vi "Main.vi"() -> ()   [LabVIEW 2019]
uses:
  <vilib>/myRIO/Instrument Drivers/Onboard IO/SPI/typedefs/SPI User Configuration.ctl
  <vilib>/myRIO/Common/Instrument Driver Framework/myRIO v1.0/SPI/typedefs/SPI Clock Phase.ctl
  <vilib>/myRIO/Common/Instrument Driver Framework/myRIO v1.0/SPI/typedefs/SPI Clock Polarity.ctl
  <vilib>/myRIO/Common/Instrument Driver Framework/myRIO v1.0/SPI/typedefs/SPI Data Direction.ctl
  <vilib>/myRIO/Common/Instrument Driver Framework/myRIO v1.0/SPI/typedefs/SPI Frame Length.ctl
  <vilib>/myRIO/Instrument Drivers/Onboard IO/AO/typedefs/AO Reference.ctl
  <vilib>/myRIO/Common/Instrument Driver Framework/Utilities/typedefs/myRIO Generic Hardware Reference.ctl
  <vilib>/myRIO/Common/Instrument Driver Framework/Utilities/typedefs/Hardware Version Enum.ctl
  <vilib>/myRIO/Common/Instrument Driver Framework/Utilities/typedefs/myRIO v1.0 Reference.ctl
  <vilib>/myRIO/Common/Instrument Driver Framework/Utilities/typedefs/Generic FPGA Reference.ctl
  <vilib>/myRIO/Common/Instrument Driver Framework/myRIO v1.0/AO/typedefs/AO Channels List.ctl
  <vilib>/myRIO/Common/Instrument Driver Framework/myRIO v1.0/AO/typedefs/AO Channels Enum.ctl
  <vilib>/myRIO/Common/Instrument Driver Framework/Utilities/typedefs/Analog Scaling Constants List.ctl
  <vilib>/myRIO/Common/Instrument Driver Framework/Utilities/typedefs/Analog Scaling Constants.ctl
  <vilib>/userdefined/High Color/nirio_resource_hc.ctl
  <vilib>/myRIO/Instrument Drivers/Onboard IO/SPI/typedefs/SPI Reference.ctl
  <vilib>/myRIO/Common/Instrument Driver Framework/myRIO v1.0/SPI/typedefs/SPI Channels Enum.ctl
  <vilib>/myRIO/Instrument Drivers/Onboard IO/SPI/typedefs/SPI Configuration.ctl
  <vilib>/myRIO/Instrument Drivers/Onboard IO/DIO/typedefs/DIO Reference.ctl
  <vilib>/myRIO/Common/Instrument Driver Framework/myRIO v1.0/DIO/typedefs/DIO Channels List.ctl
  <vilib>/myRIO/Common/Instrument Driver Framework/myRIO v1.0/DIO/typedefs/DIO Channels Enum.ctl
  <vilib>/Platform/TimedLoop/XDataNode/timing_clust.ctl
  <vilib>/Platform/TimedLoop/XDataNode/nitl_modes.ctl
  <vilib>/Platform/TimedLoop/XDataNode/wakeup.ctl
  <vilib>/myRIO/Instrument Drivers/Onboard IO/AI/typedefs/AI Reference.ctl
  <vilib>/myRIO/Common/Instrument Driver Framework/myRIO v1.0/AI/typedefs/AI Channels List.ctl
  <vilib>/myRIO/Common/Instrument Driver Framework/myRIO v1.0/AI/typedefs/AI Channels Enum.ctl
  <vilib>/Analysis/3filter.llb/Filter Passband Type.ctl
  <vilib>/myRIO/Instrument Drivers/Onboard IO/PWM/typedefs/PWM Reference.ctl
  <vilib>/myRIO/Common/Instrument Driver Framework/myRIO v1.0/PWM/typedefs/PWM Channels Enum.ctl
  <vilib>/myRIO/Instrument Drivers/Onboard IO/PWM/typedefs/PWM Configuration.ctl
  <vilib>/myRIO/Common/Instrument Driver Framework/Utilities/vis/Is FPGA Ref Available.vi
  <vilib>/myRIO/Common/Instrument Driver Framework/myRIO v1.0/AO/vis/myRIO v1.1 Open AO.vi
  <vilib>/myRIO/Instrument Drivers/Onboard IO/AO/vis/Write.vi
  <vilib>/myRIO/Common/Instrument Driver Framework/myRIO v1.0/SPI/vis/myRIO v1.1 Open SPI.vi
  <vilib>/myRIO/Common/Instrument Driver Framework/myRIO v1.0/DIO/vis/myRIO v1.1 Open DIO.vi
  <vilib>/myRIO/Instrument Drivers/Onboard IO/DIO/vis/Write.vi
  <vilib>/myRIO/Common/Instrument Driver Framework/myRIO v1.0/AI/vis/myRIO v1.1 Open AI.vi
  <vilib>/myRIO/Instrument Drivers/Onboard IO/AI/vis/Read.vi
  <vilib>/myRIO/Common/Instrument Driver Framework/myRIO v1.0/PWM/vis/myRIO v1.1 Open PWM.vi
  <vilib>/myRIO/Instrument Drivers/Onboard IO/PWM/vis/Set Duty Cycle and Frequency.vi
  <vilib>/myRIO/Common/Instrument Driver Framework/Utilities/vis/Validate Channels.vi
  <vilib>/myRIO/Common/Instrument Driver Framework/myRIO v1.0/AO/vis/myRIO v1.0 Reserve AO.vi
  <vilib>/myRIO/Common/Instrument Driver Framework/myRIO v1.0/SPI/vis/myRIO v1.0 Reserve SPI.vi
  <vilib>/myRIO/Common/Instrument Driver Framework/myRIO v1.0/DIO/vis/myRIO v1.0 Reserve DIO.vi
  <vilib>/myRIO/Common/Instrument Driver Framework/myRIO v1.0/AI/vis/myRIO v1.0 Reserve AI.vi
  <vilib>/myRIO/Common/Instrument Driver Framework/myRIO v1.0/PWM/vis/myRIO v1.0 Reserve PWM.vi
  <vilib>/myRIO/Common/Instrument Driver Framework/myRIO v1.0/SPI/vis/myRIO v1.0 Close SPI.vi
  <vilib>/myRIO/Common/Instrument Driver Framework/myRIO v1.0/UART/vis/myRIO v1.0 Close UART.vi
  <vilib>/myRIO/Common/Instrument Driver Framework/myRIO v1.0/AO/vis/myRIO v1.0 Build MUX Configuration AO.vi
  <vilib>/myRIO/Common/Instrument Driver Framework/myRIO v1.0/Resource Manager/vis/myRIO v1.0 Reserve Channel List.vi
  <vilib>/myRIO/Common/Instrument Driver Framework/myRIO v1.0/SPI/vis/myRIO v1.0 Build MUX Configuration SPI.vi
  <vilib>/myRIO/Common/Instrument Driver Framework/myRIO v1.0/DIO/vis/myRIO v1.0 Build MUX Configuration DIO.vi
  <vilib>/myRIO/Common/Instrument Driver Framework/myRIO v1.0/AI/vis/myRIO v1.0 Build MUX Configuration AI.vi
  <vilib>/myRIO/Common/Instrument Driver Framework/myRIO v1.0/PWM/vis/myRIO v1.0 Build MUX Configuration PWM.vi
  <vilib>/myRIO/Common/Instrument Driver Framework/myRIO v1.0/SPI/vis/myRIO v1.0 Unreserve SPI.vi
  <vilib>/myRIO/Common/Instrument Driver Framework/myRIO v1.0/Resource Manager/vis/myRIO v1.0 Reserve Channel.vi
  <vilib>/myRIO/Common/Instrument Driver Framework/myRIO v1.0/Resource Manager/vis/myRIO v1.0 Unreserve Channel.vi
  <vilib>/myRIO/Common/Instrument Driver Framework/myRIO v1.0/Resource Manager/vis/myRIO v1.0 Create Configuration List.vi
  <vilib>/myRIO/Common/Instrument Driver Framework/myRIO v1.0/Resource Manager/vis/myRIO v1.0 Unreserve Channel List.vi
  <vilib>/myRIO/Common/Instrument Driver Framework/myRIO v1.0/Resource Manager/vis/myRIO v1.0 Build Mutex Name.vi
  <vilib>/Utility/VariantDataType/GetNumericInfo.vi
  <vilib>/Utility/error.llb/Error Cluster From Error Code.vi
  <vilib>/myRIO/Common/Instrument Driver Framework/myRIO v1.0/myRIO v1.1 Open.vi
  <vilib>/myRIO/Common/Instrument Driver Framework/Utilities/vis/IO Manager.vi
  <vilib>/myRIO/Common/Instrument Driver Framework/Utilities/vis/Configuration Manager.vi
  <vilib>/myRIO/Common/Instrument Driver Framework/myRIO v1.0/Resource Manager/vis/myRIO v1.0 Configure IO.vi
  <vilib>/myRIO/Common/Instrument Driver Framework/myRIO v1.0/myRIO v1.0 Close.vi
  <vilib>/myRIO/Common/Instrument Driver Framework/myRIO v1.0/DIO/vis/myRIO v1.0 Write DIO.vi
  <vilib>/myRIO/Common/Instrument Driver Framework/myRIO v1.0/SPI/vis/myRIO v1.0 Configure SPI.vi
  <vilib>/myRIO/Common/Instrument Driver Framework/myRIO v1.0/AO/vis/myRIO v1.0 Get Scaling Constants AO.vi
  <vilib>/myRIO/Common/Instrument Driver Framework/myRIO v1.0/AO/vis/myRIO v1.0 Write AO.vi
  <vilib>/myRIO/Common/Instrument Driver Framework/myRIO v1.0/AI/vis/myRIO v1.0 Get Scaling Constants AI.vi
  <vilib>/myRIO/Common/Instrument Driver Framework/myRIO v1.0/AI/vis/myRIO v1.0 Read AI.vi
  <vilib>/functionblocks/Edge Detection/One Shot Rising with Input/One Shot Rising with Input.vi
  <vilib>/myRIO/Common/Instrument Driver Framework/myRIO v1.0/PWM/vis/myRIO v1.0 Write PWM.vi
  <vilib>/myRIO/Common/Instrument Driver Framework/myRIO v1.0/SPI/vis/myRIO v1.0 Shutdown SPI.vi
  <vilib>/myRIO/Common/Instrument Driver Framework/Utilities/vis/FPGA Ref Manager.vi
  <vilib>/myRIO/Common/Instrument Driver Framework/myRIO v1.0/myRIO v1.0 Reset FPGA.vi
  <vilib>/myRIO/Common/Instrument Driver Framework/myRIO v1.0/IRQ/vis/myRIO v1.0 IRQ Info FGV.vi
  <vilib>/myRIO/Common/Instrument Driver Framework/myRIO v1.0/IRQ/vis/myRIO v1.0 Timer IRQ Info FGV.vi
  <vilib>/myRIO/Common/Instrument Driver Framework/myRIO v1.0/IRQ/vis/myRIO v1.0 ISR Agent.vi
  <vilib>/myRIO/Instrument Drivers/Utilities/vis/Reset Index.vi
  <vilib>/myRIO/Common/Instrument Driver Framework/myRIO v1.0/Resource Manager/vis/myRIO v1.0 Block Write Resource Manager.vi
  <vilib>/myRIO/Express VI/Onboard IO/DO/DO Express VI.xnode
  <vilib>/myRIO/Instrument Drivers/Onboard IO/DIO/vis/myRIO DIO Open.xnode
  <vilib>/myRIO/Instrument Drivers/Onboard IO/SPI/vis/myRIO SPI Open.xnode
  <vilib>/myRIO/Express VI/Onboard IO/AO/AO Express VI.xnode
  <vilib>/myRIO/Instrument Drivers/Onboard IO/AO/vis/myRIO AO Open.xnode
  <vilib>/Platform/TimedLoop/XDataNode/XDataNode.xnode
  <vilib>/myRIO/Express VI/Onboard IO/AI/AI Express VI.xnode
  <vilib>/myRIO/Instrument Drivers/Onboard IO/AI/vis/myRIO AI Open.xnode
  <vilib>/functionblocks/FB Core/FB Core.xnode
  <vilib>/regexp/Match Regular Expression.xnode
  <vilib>/myRIO/Express VI/Onboard IO/PWM/PWM Express VI.xnode
  <vilib>/myRIO/Instrument Drivers/Onboard IO/PWM/vis/myRIO PWM Open.xnode
  <vilib>/myRIO/Instrument Drivers/Utilities/Utilities.lvlib
  <vilib>/myRIO/Instrument Drivers/Onboard IO/SPI/SPI.lvlib
  <vilib>/myRIO/Instrument Drivers/Onboard IO/AI/AI.lvlib
  <vilib>/Platform/TimedLoop/XDataNode/XDNodeRunTimeDep.lvlib
  <vilib>/myRIO/Instrument Drivers/Onboard IO/DIO/DIO.lvlib
  <vilib>/myRIO/Instrument Drivers/Onboard IO/PWM/PWM.lvlib
  <vilib>/myRIO/Instrument Drivers/Onboard IO/AO/AO.lvlib
  <vilib>/functionblocks/NI_FunctionBlock Libraries.lvlib
  <vilib>/ptbypt/NI_PtbyPt.lvlib
  <vilib>/Analysis/NI_AALBase.lvlib
panel:
  in  "Leg Length":dbl=1.0
  out "Speed":cluster{"Numeric":dbl, dbl}(graph)
  in  "Controller":enum16{"ML", "TBE"}(ring)
  out "size(s)":i32
  in  "SEND DATA !!\nLETS GO!":bool
  out "R.FSR":bool
  out "L.FSR":bool
  out "True Walking Speed":dbl=0.1 format="%#_13g"
  out "Assistant Profile":cluster{dbl, dbl}(graph)
  in  "Torque GO!":bool
  out "Trunk IMU":T1(graph)
  out "Right IMU":T1(graph)
  in  "Body Weight":dbl
  in  "Hip Angle Init":bool
  out "SYNC":bool
  in  "Assist":bool
  out "L.Limit":bool
  out "R.Limit":bool
  out "Left Torque":T2(graph)
  in  "Saving File Name":string
  out "Hip Angle":cluster{dbl, dbl}(graph)
  out "Right Torque":T3(graph)
  out "Run Time":dbl
  in  "Motor Enable":bool
  out "Loop Time":u32
  in  "STOP":bool
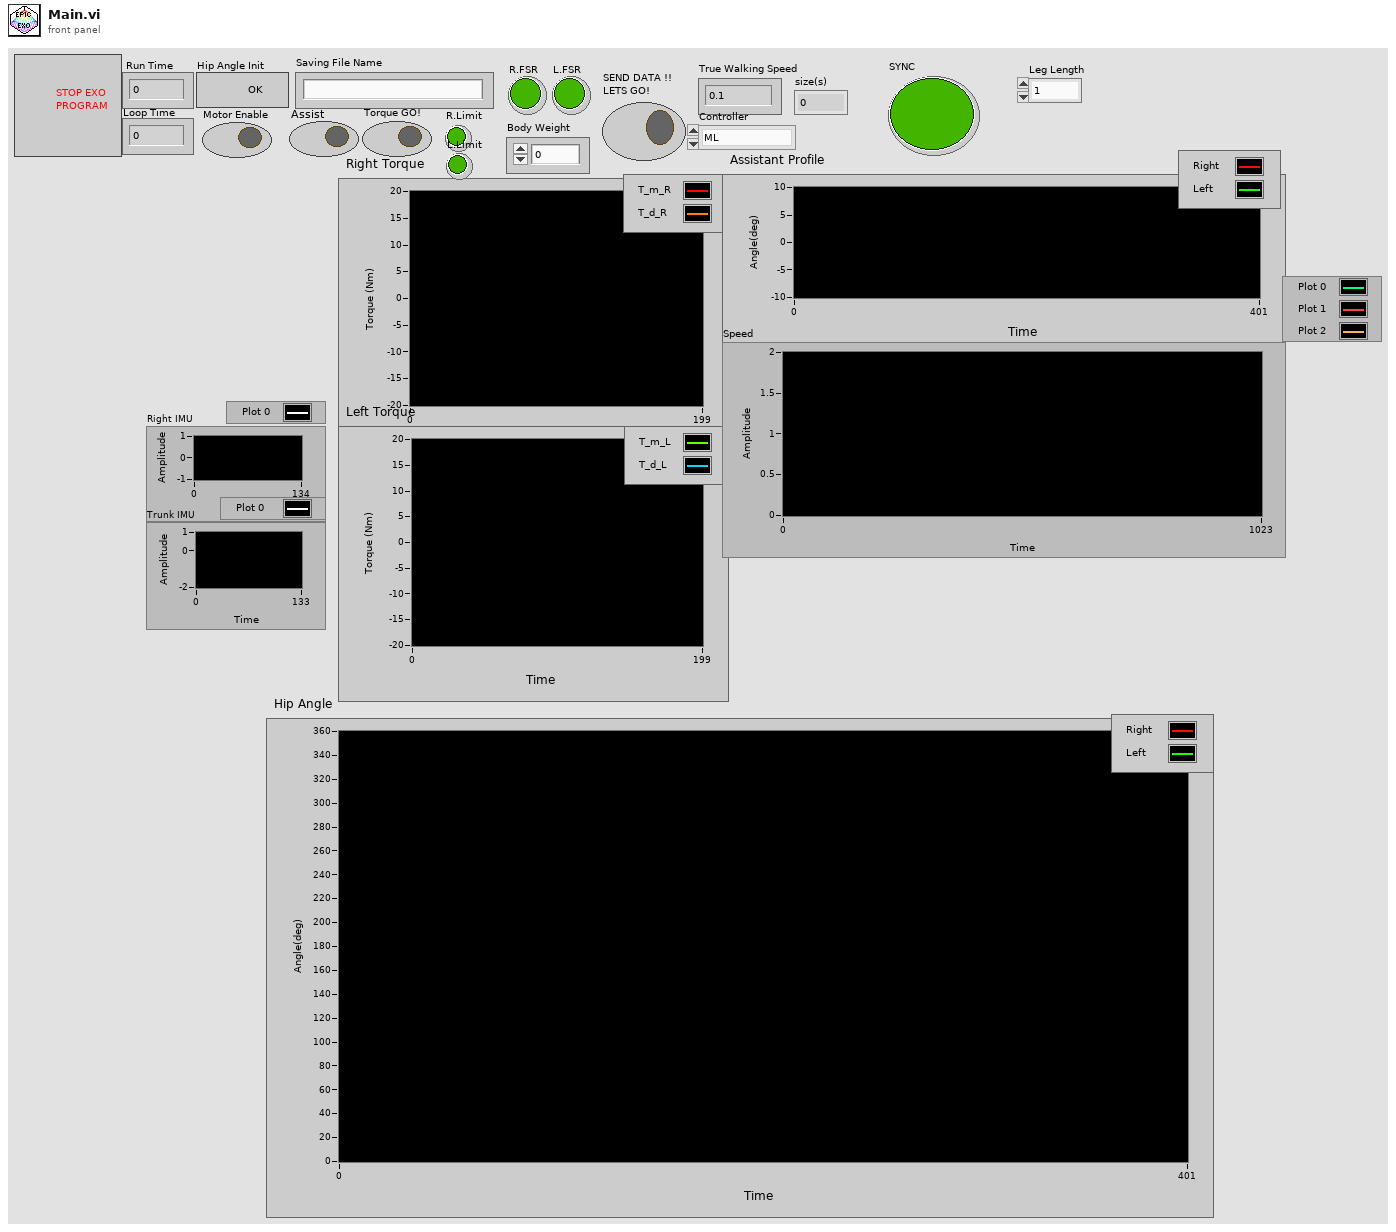
[diagram p1: front panel]
types:
  T1 = cluster{"[0]":dbl, "[1]":dbl, "[2]":dbl, "[3]":dbl, "[4]":dbl, "[5]":dbl, "[6]":dbl, "[7]":dbl, "[8]":dbl}
  T2 = cluster{"Left Torque":dbl, "Left Desired Torque":dbl}
  T3 = cluster{"Right Torque in":dbl, "Right Torque Desired":dbl}
  T4 = typedef "SPI.lvlib/SPI User Configuration.ctl" = cluster{"Frequency [Hz]":dbl, "Clock Phase":T5, "Clock Polarity":T6, "Data Direction":T7, "Frame Length":T8}
  T5 = typedef "SPI Clock Phase.ctl" = enum8{"Leading", "Trailing"}
  T6 = typedef "SPI Clock Polarity.ctl" = enum8{"Low", "High"}
  T7 = typedef "SPI Data Direction.ctl" = enum8{"Most significant bit first", "Least significant bit first"}
  T8 = typedef "SPI Frame Length.ctl" = u8
  T9 = typedef "AO.lvlib/AO Reference.ctl" = cluster{"myRIO Reference":T10, "AO Channel List":T14, "AO Scaling Constant List":T16}
  T10 = typedef "myRIO Generic Hardware Reference.ctl" = cluster{"myRIO Model":T11, "myRIO Hardware Reference":T12}
  T11 = typedef "Hardware Version Enum.ctl" = enum16{"Unknown", "myRIO-1900", "myRIO-1950", "roboRIO", "NI ELVIS RIO CM", "ELVIS III"}
  T12 = typedef "myRIO v1.0 Reference.ctl" = cluster{"Generic FPGA Reference":T13, "Allow multiple opens":bool}
  T13 = typedef "Generic FPGA Reference.ctl" = refnum<k20>
  T14 = typedef "AO Channels List.ctl" = T15[]
  T15 = typedef "AO Channels Enum.ctl" = enum16{"Not Connected", "AudioOut/Left", "AudioOut/Right", "C/AO0", "C/AO1", "A/AO0", "A/AO1", "B/AO0", "B/AO1"}
  T16 = typedef "Analog Scaling Constants List.ctl" = T17[]
  T17 = typedef "Analog Scaling Constants.ctl" = cluster{"LSB Weight (Volts)":dbl, "Offset (Volts)":dbl, "Signed?":bool}
  T18 = typedef "nirio_resource_hc.ctl" = tag
  T19 = typedef "DIO.lvlib/DIO Reference.ctl" = cluster{"myRIO Reference":T10, "DIO Channels List":T20}
  T20 = typedef "DIO Channels List.ctl" = T21[]
  T21 = typedef "DIO Channels Enum.ctl" = enum16{"Not Connected", "C/DIO0", "C/DIO1", "C/DIO2", "C/DIO3", "C/DIO4", "C/DIO5", "C/DIO6", "C/DIO7", "A/DIO0", "A/DIO1", "A/DIO2", "A/DIO3", "A/DIO4", "A/DIO5", "A/DIO6", "A/DIO7", "A/DIO8", "A/DIO9", "A/DIO10", "A/DIO11", "A/DIO12", "A/DIO13", "A/DIO14", "A/DIO15", "A/DIO16", "A/DIO17", "A/DIO18", "A/DIO19", "B/DIO0", "B/DIO1", "B/DIO2", "B/DIO3", "B/DIO4", "B/DIO5", "B/DIO6", "B/DIO7", "B/DIO8", "B/DIO9", "B/DIO10", "B/DIO11", "B/DIO12", "B/DIO13", "B/DIO14", "B/DIO15", "B/DIO16", "B/DIO17", "B/DIO18", "B/DIO19", "LED0", "LED1", "LED2", "LED3", "Button0", "DIO/DIO0", "DIO/DIO1", "DIO/DIO2", "DIO/DIO3", "DIO/DIO4", "DIO/DIO5", "DIO/DIO6", "DIO/DIO7", "DIO/DIO8", "DIO/DIO9", "SPI/CS0", "SPI/CS1", "SPI/CS2", "SPI/CS3", "LED RADIO (Green)", "LED RADIO (Red)", "LED COMM (Green)", "LED COMM (Red)", "LED MODE (Green)", "LED MODE (Red)"}
  T22 = typedef "AI.lvlib/AI Reference.ctl" = cluster{"myRIO Reference":T10, "AI Channels List":T23, "AI Scaling Constants List":T16}
  T23 = typedef "AI Channels List.ctl" = T24[]
  T24 = typedef "AI Channels Enum.ctl" = enum16{"Not Connected", "AudioIn/Left", "AudioIn/Right", "C/AI0", "C/AI1", "A/AI0", "A/AI1", "A/AI2", "A/AI3", "A/AI4", "A/AI5", "A/AI6", "A/AI7", "B/AI0", "B/AI1", "B/AI2", "B/AI3", "B/AI4", "B/AI5", "B/AI6", "B/AI7", "AI/AI0", "AI/AI1", "AI/AI2", "AI/AI3", "A/AI0 (DIFF)", "A/AI1 (DIFF)", "A/AI2 (DIFF)", "A/AI3 (DIFF)", "B/AI0 (DIFF)", "B/AI1 (DIFF)", "B/AI2 (DIFF)", "B/AI3 (DIFF)"}
  T25 = typedef "XDNodeRunTimeDep.lvlib/timing_clust.ctl" = cluster{"Expected End [f-1]":u64, "Actual End [f-1]":u64, "Finished Late? [f-1]":bool, "Expected End [i-1]":u64, "Actual End [i-1]":u64, "Finished Late? [i-1]":bool, "Expected Start [i]":u64, "Actual Start [i]":u64, "Expected Start [f]":u64, "Actual Start [f]":u64, "Source Name":string, "Structure Name":string, "Period":i64, "Deadline":i64, "Offset":i64, "Start":i64, "Priority":i32, "Timeout":i32, "Mode":T26, "Wakeup Reason":T27, "Error":errorcluster, "Source Type":string, "Secondary Source Type":string, "Global End Time":u64, "Global Start Time":u64, "Frame Duration":u64, "Iteration Duration":u64, "Assigned CPU":i32, "I/O Scan Engine Mode":u32}
  T26 = typedef "XDNodeRunTimeDep.lvlib/nitl_modes.ctl" = enum32{"No Change", "Process missed periods, maintain original phase", "Discard missed periods, maintain original phase", "Process missed periods, ignore original phase", "Discard missed periods, ignore original phase"}
  T27 = typedef "XDNodeRunTimeDep.lvlib/wakeup.ctl" = enum32{"Normal", "Aborted", "Asynchronous wakeup", "Timing source error", "Timed loop error", "Timeout"}
  T28 = enum16{"Standard", "Buffered", "CRLF", "Immediate"}
  T29 = typedef "NI_AALBase.lvlib/Filter Passband Type.ctl" = enum32{"Lowpass", "Highpass", "Bandpass", "Bandstop"}
  T30 = typedef "PWM.lvlib/PWM Reference.ctl" = cluster{"myRIO Reference":T10, "PWM Channels Enum":T31, "PWM Configuration":T32}
  T31 = typedef "PWM Channels Enum.ctl" = enum16{"Not Connected", "C/PWM0", "C/PWM1", "A/PWM0", "A/PWM1", "A/PWM2", "A/PWM3", "A/PWM4", "A/PWM5", "A/PWM6", "A/PWM7", "A/PWM8", "A/PWM9", "A/PWM10", "A/PWM11", "A/PWM12", "A/PWM13", "A/PWM14", "A/PWM15", "A/PWM16", "A/PWM17", "A/PWM18", "A/PWM19", "B/PWM0", "B/PWM1", "B/PWM2", "B/PWM3", "B/PWM4", "B/PWM5", "B/PWM6", "B/PWM7", "B/PWM8", "B/PWM9", "B/PWM10", "B/PWM11", "B/PWM12", "B/PWM13", "B/PWM14", "B/PWM15", "B/PWM16", "B/PWM17", "B/PWM18", "B/PWM19", "PWM/PWM0", "PWM/PWM1", "PWM/PWM2", "PWM/PWM3", "PWM/PWM4", "PWM/PWM5", "PWM/PWM6", "PWM/PWM7", "PWM/PWM8", "PWM/PWM9"}
  T32 = typedef "PWM.lvlib/PWM Configuration.ctl" = cluster{"Frequency":dbl, "Duty Cycle":dbl}
  T33 = typedef "SPI.lvlib/SPI Reference.ctl" = cluster{"myRIO Reference":T10, "SPI Channels Enum":T34, "SPI Configuration":T35}
  T34 = typedef "SPI Channels Enum.ctl" = enum16{"Not Connected", "A/SPI", "B/SPI", "SPI/SPI"}
  T35 = typedef "SPI.lvlib/SPI Configuration.ctl" = cluster{"Frequency [Hz]":dbl, "Clock Phase":T5, "Clock Polarity":T6, "Data Direction":T7, "Frame Length":T8}
  T36 = cluster{"Torque Output":dbl, "Torque Output":dbl}
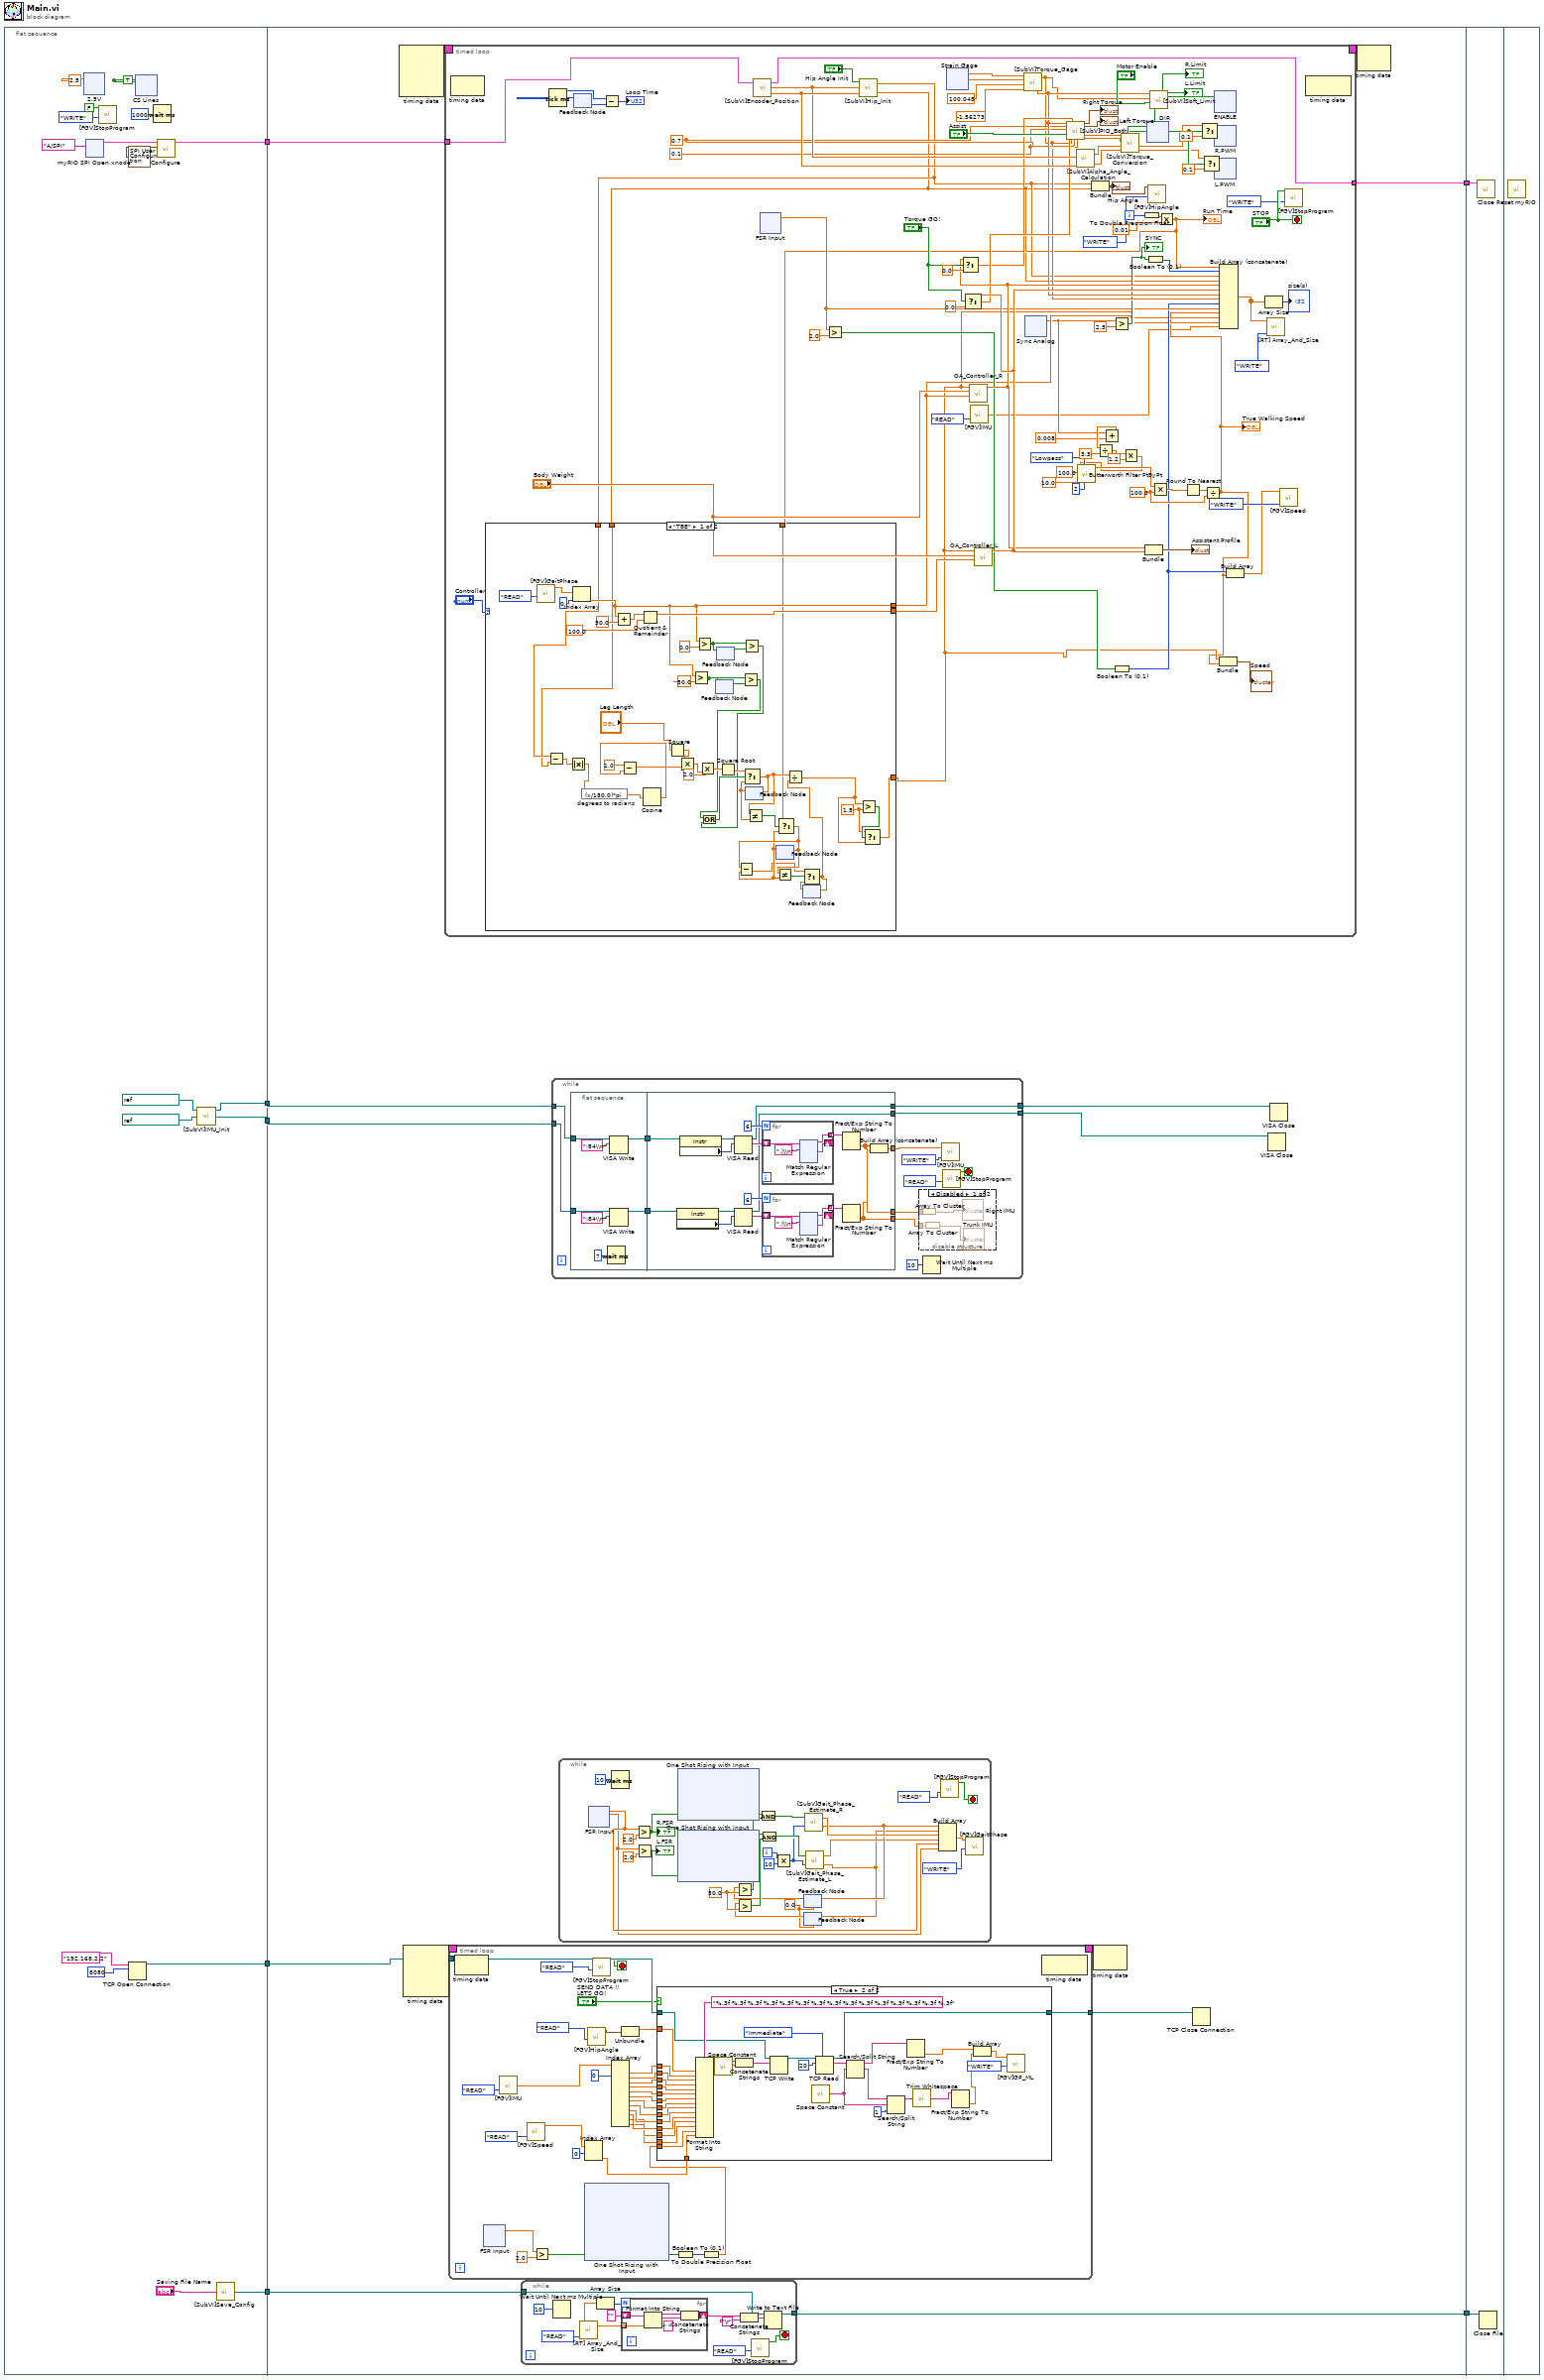
[diagram p0: block diagram]
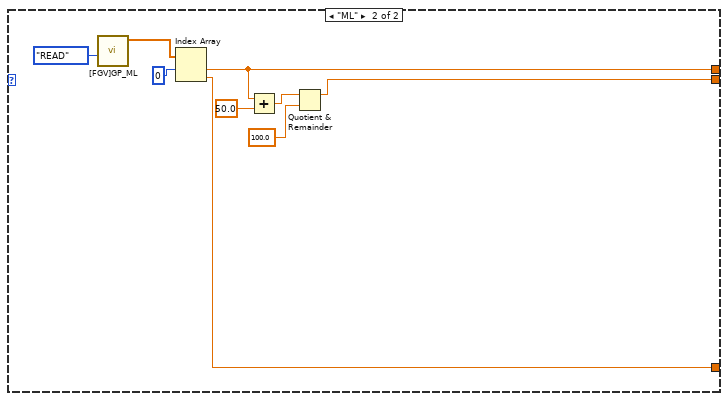
[diagram p4: hidden frame]
diagram:
  n1 = flat-sequence {
    tunnel: [w20] -> w7
    tunnel: [w18] -> w4
    tunnel: [w9] -> w3
    tunnel: [w8] -> w2
    tunnel: [w12] -> w1
    tunnel: w7 -> [w126]
    tunnel: [w125] -> w6
    tunnel: [w124] -> w5
    tunnel: w4 -> [w123]
    tunnel: w3 -> [w120]
    tunnel: w2 -> [w119]
    tunnel: w1 -> [w117]
    tunnel: w6 -> [w1117]
    tunnel: w5 -> [w1116]
    frame #0 {
      w16 = TRUE ("A/DIO2 (Pin 15)")
      n2 = xnode "2.5V"("2.5V (B/AO0 (Pin 2))"=2.5 ("2.5V (A/AO0 (Pin 2))")) -> ()  [unwired: 1 in, 1 out]
      n3 = xnode "myRIO SPI Open.xnode"("Channel Name"=tag "A/SPI") -> ("SPI Ref Out"=w23:T33)  [unwired: 2 in, 1 out]
      n4 = call "[FGV]StopProgram.vi"("Select"=enum16{"READ", "WRITE"}."WRITE", "Flag In"=FALSE) -> ()  [unwired: 9 in, 1 out]
      n5 = TCP Open Connection(address="192.168.2.2", remote port or service name=u16 8080) -> (connection ID=w12:refnum<k5>)  [unwired: 3 in, 1 out]
      n6 = xnode "CS Lines"("cs1 (A/DIO14 (Pin 32))"=w16, "cs2 (A/DIO15 (Pin 34))"=w16) -> ()  [unwired: 1 in, 1 out]
      n7 = Wait (ms)(milliseconds to wait=u32 1000) -> ()  [unwired: 1 out]
      n8 = call <vilib>:"Configure.vi"("SPI User Configuration"=T4 {"Frequency [Hz]"=4000000.0, "Clock Phase"=enum."Trailing", "Clock Polarity"=enum."Low", "Data Direction"=enum."Most significant bit first", "Frame Length"=8}, "SPI Ref In"=w23) -> ("SPI Ref Out"=w20:T33)  [unwired: 8 in, 1 out]
      n9 = call "[SubVI]IMU_Init.vi"("IMU Left"=refnum<visa-resource-name> "ASRL4::INSTR" ("VISA resource name"), "IMU Thigh"=refnum<visa-resource-name> "ASRL5::INSTR" ("VISA resource name")) -> ("IMU Left Out"=w8:refnum<visa-resource-name>, "IMU Right Out"=w9:refnum<visa-resource-name>)  [unwired: 1 in, 1 out]
      n10 = call "[SubVI]Save_Config.vi"("Saving File Name"="Saving File Name") -> ("Byte Stream File out"=w18:refnum<file>)
    }
    frame #1 {
      n11 = node-c288() -> (w128:T25)  [unwired: 4 in]
      n12 = node-c288() -> (w116:T25)  [unwired: 4 in]
      n13 = timed-loop {
        timing: w128 -> [_]
        timing-out: [_] -> w127
        tunnel: w126 -> [w781]
        tunnel: [w799] -> w125
        i -> [w776]
        stop <- "STOP" stop-if-true
        w751 = 100.0 ("y")
        w757 = 0.7 ("kp_right")
        w756 = 0.1 ("kd_right")
        n14 = node-c288() -> ()  [unwired: 1 in, 1 out]
        n15 = Tick Count (ms)() -> (millisecond timer value=w795:u32)
        n16 = feedback-in #1(w795) -> ()
        n17 = feedback #1() -> (w794:u32)  [unwired: 1 in]
        n18 = Subtract(x=w795, y=w794) -> (x-y=→"Loop Time":u32)
        n19 = call "[SubVI]Encoder_Position.vi"("SPI Reference In in"=w781) -> ("Left Theta"=w767:dbl, "Right Theta"=w766:dbl, "SPI Reference In out"=w799:T33)  [unwired: 2 out]
        n20 = xnode "FSR Input"() -> ("FSR 1 - Right (B/AI0 (Pin 3))"=w738:dbl)  [unwired: 1 in, 2 out]
        n21 = Greater?(x=w738, y=2.0) -> (0:w736:bool)
        n22 = call "[SubVI]Hip_Init.vi"("Left Theta"=w767, "Right Theta"=w766, "Hip Init"="Hip Angle Init") -> ("Left Hip"=w730:dbl, "Right Hip"=w731:dbl)
        n23 = xnode "Strain Gage"() -> ("Right (B/AI2 (Pin 7))"=w788:dbl, "Left (B/AI3 (Pin 9))"=w787:dbl)  [unwired: 1 in, 1 out]
        n24 = call "[FGV]IMU.vi"("Select"=enum16{"READ", "WRITE"}."READ") -> ("IMU Out"=w714:dbl[])  [unwired: 1 in]
        n25 = call "[SubVI]Torque_Gage.vi"("Left Offset"=-1.56273 ("Right Offset"), "Right Offset"=100.045, "Left Input"=w787, "Right Input"=w788) -> ("Right Torque"=w758:dbl, "Left Torque"=w754:dbl)
        n26 = xnode "Sync Analog"() -> ("A/AI0 (Pin 3)"=w720:dbl)  [unwired: 1 in, 1 out]
        n27 = call "[SubVI]Alpha_Angle_Calculation.vi"("Left Theta"=w767, "Right Theta"=w766) -> ("Left Alpha"=w764:dbl, "Right Alpha"=w765:dbl)  [unwired: 2 in]
        n28 = Bundle("Right Hip"=w731, "Left Hip"=w730) -> (w769:cluster{"Right Hip":dbl, "Left Hip":dbl})  [unwired: 1 in]
        "Hip Angle" <- w769
        n29 = Add(x=w720, y=0.008) -> (x+y=w721:dbl)
        n30 = Divide(x=w721, y=3.3) -> (x/y=w723:dbl)
        n31 = Greater?(x=w720, y=2.5) -> (0:w749:bool)
        "SYNC" <- w749
        n32 = Boolean To (0,1)(Boolean=w736) -> (0, 1=w735:i16)
        n33 = Multiply(x=w723, y=1.2) -> (x*y=w719:dbl)
        n34 = call <vilib>:"Butterworth Filter PtByPt.vi"("order"=2, "filter type"=Filter_Passband_Type."Lowpass", "low cutoff freq: fl"=10.0, "sampling freq: fs"=100.0, "x"=w719) -> ("Filtered x"=w725:dbl)  [unwired: 4 in, 1 out]
        n35 = To Double Precision Float(number=w776) -> (double precision float=w790:dbl)
        n36 = Boolean To (0,1)(Boolean=w749) -> (0, 1=w792:i16)
        n37 = call "[FGV]HipAngle.vi"("Select"=enum16{"READ", "WRITE"}."WRITE", "Hip In"=w769) -> ()  [unwired: 9 in, 1 out]
        n38 = call "[SubVI]Soft_Limit.vi"("Motor Enable in"="Motor Enable", "Left Torque"=w754, "Right Torque"=w758) -> ("PWM out"=w783:bool, "ENA out"=w782:bool, "L.SLimit"=→"L.Limit":bool, "R.SLimit"=→"R.Limit":bool)  [unwired: 1 in]
        n39 = Multiply(x=w725, y=w751) -> (x*y=w753:dbl)
        n40 = Multiply(x=w790, y=0.01) -> (x*y=w732:dbl)
        "Run Time" <- w732
        n41 = case shown="\"TBE\"" "Controller" {
          tunnel: [w839 w850] -> w733
          tunnel: [w842 w851] -> w734
          tunnel: w732 -> [w810 _]
          tunnel: [w804 w849] -> w716
          tunnel: w731 -> [w809 _]
          tunnel: w730 -> [w808 _]
          frame "TBE" {
            w806 = 1.5 ("y")
            n42 = call "[FGV]GaitPhase.vi"("Select"=enum16{"READ", "WRITE"}."READ") -> ("GP Out"=w847:dbl[])  [unwired: 10 in]
            n43 = Subtract(x=w809, y=w808) -> (x-y=w834:dbl)
            n44 = Absolute Value(x=w834) -> (abs(x)=w832:dbl)
            n45 = Index Array(array=w847, index=0) -> (element=w839:dbl)
            n46 = expression code="(x/180.0)*pi" "degrees to radians"(w832) -> (w831:dbl)
            n47 = Add(x=w839, y=50.0) -> (x+y=w844:dbl)
            n48 = Quotient & Remainder(x=w844, y=100.0) -> (x-y*floor(x/y)=w842:dbl)  [unwired: 1 out]
            n49 = Cosine(x=w831) -> (cos(x)=w830:dbl)
            n50 = Subtract(x=1.0, y=w830) -> (x-y=w829:dbl)
            n51 = Square(x="Leg Length") -> (x^2=w828:dbl)
            n52 = Multiply(x=w828, y=w829) -> (x*y=w827:dbl)
            n53 = Greater?(x=w839, y=50.0) -> (0:w835:bool)
            n54 = Greater?(x=w839, y=0.0) -> (0:w837:bool)
            n55 = Multiply(x=2.0, y=w827) -> (x*y=w825:dbl)
            n56 = feedback #2() -> (w836:bool)  [unwired: 1 in]
            n57 = feedback-in #2(w835) -> ()
            n58 = feedback-in #3(w837) -> ()
            n59 = feedback #3() -> (w838:bool)  [unwired: 1 in]
            n60 = Square Root(x=w825) -> (sqrt(x)=w813:dbl)
            n61 = Greater?(x=w835, y=w836) -> (0:w812:bool)
            n62 = Greater?(x=w837, y=w838) -> (0:w811:bool)
            n63 = Or(x=w812, y=w811) -> (x .or. y?=w814:bool)
            n64 = feedback #4() -> (w823:dbl)  [unwired: 1 in]
            n65 = Select(t=w813, s=w814, f=w823) -> (s? t:f=w815:dbl)
            n66 = feedback-in #4(w815) -> ()
            n67 = Not Equal?(x=w815, y=w823) -> (x != y?=w822:bool)
            n68 = feedback #5() -> (w820:dbl)  [unwired: 1 in]
            n69 = Select(t=w810, s=w822, f=w820) -> (s? t:f=w821:dbl)
            n70 = Subtract(x=w821, y=w820) -> (x-y=w818:dbl)
            n71 = feedback-in #5(w821) -> ()
            n72 = Not Equal?(x=w821, y=w820) -> (x != y?=w819:bool)
            n73 = feedback #6() -> (w817:dbl)  [unwired: 1 in]
            n74 = Select(t=w818, s=w819, f=w817) -> (s? t:f=w816:dbl)
            n75 = Divide(x=w815, y=w816) -> (x/y=w805:dbl)
            n76 = feedback-in #6(w816) -> ()
            n77 = Greater?(x=w805, y=w806) -> (0:w807:bool)
            n78 = Select(t=w806, s=w807, f=w805) -> (s? t:f=w804:dbl)
          }
          frame "ML" {
            n79 = call "[FGV]GP_ML.vi"("Select"=enum16{"READ", "WRITE"}."READ") -> ("GP Out"=w852:dbl[])  [unwired: 10 in]
            n80 = Index Array(array=w852, index #1=0 ("index")) -> (element #1=w850:dbl, element #2=w849:dbl)  [unwired: 1 in]
            n81 = Add(x=w850, y=50.0) -> (x+y=w854:dbl)
            n82 = Quotient & Remainder(x=w854, y=100.0) -> (x-y*floor(x/y)=w851:dbl)  [unwired: 1 out]
          }
        }
        n83 = call "OA_Controller_R.vi"("Gait Phase"=w733, "Weight"="Body Weight", "Walking Speed"=w716) -> ("Torque Output"=w770:dbl)  [unwired: 8 in]
        n84 = Select(t=w770, s="Torque GO!", f=0.0) -> (s? t:f=w759:dbl)
        n85 = call "OA_Controller_L.vi"("Gait Phase"=w734, "Weight"="Body Weight", "Walking Speed"=w716) -> ("Torque Output"=w771:dbl)  [unwired: 8 in]
        n86 = Select(t=w771, s="Torque GO!", f=0.0) -> (s? t:f=w760:dbl)
        n87 = call "[SubV]PID_Both.vi"("Right Torque in"=w758, "Kp_left"=w757, "Kd_left"=w756, "Assist"="Assist", "Left Torque Desired"=w760, "Right Torque Desired"=w759, "Left Torque in"=w754, "kp_right"=w757, "kd_right"=w756) -> ("Right Torque"=→"Right Torque":T3, "Left Torque"=→"Left Torque":T2, "Right T Command"=w747:dbl, "Left T Command"=w746:dbl)  [unwired: 7 in]
        n88 = call "[SubVI]Torque_Conversion.vi"("Left Alpha Angle"=w764, "Right Alpha Angle"=w765, "Left Torque In"=w746, "Right Torque In"=w747) -> ("Left PWM"=w744:dbl, "Right PWM"=w745:dbl, "Left DIR"=w777:bool, "Right DIR"=w778:bool)  [unwired: 2 out]
        n89 = Bundle("Torque Output"=w770, "Torque Output"=w771) -> (→"Assistant Profile":T36)  [unwired: 1 in]
        n90 = xnode "DIR"("Right DIR (A/DIO4 (Pin 19))"=w778, "Left DIR (A/DIO8 (Pin 27))"=w777) -> ()  [unwired: 1 in, 1 out]
        n91 = Round To Nearest(number=w753) -> (nearest integer value=w752:dbl)
        n92 = Select(t=w745, s=w783, f=0.1) -> (s? t:f=w796:dbl)
        n93 = Select(t=w744, s=w783, f=0.1) -> (s? t:f=w797:dbl)
        n94 = Divide(x=w752, y=w751) -> (x/y=w715:dbl)
        "True Walking Speed" <- w715
        n95 = xnode "ENABLE"("ENABLE (A/DIO3 (Pin 17))"=w782) -> ()  [unwired: 1 in, 1 out]
        n96 = xnode "R.PWM"("Duty Cycle"=w796) -> ()  [unwired: 1 in, 1 out]
        n97 = xnode "L.PWM"("Duty Cycle"=w797) -> ()  [unwired: 1 in, 1 out]
        n98 = Bundle("Numeric"=w716, w715) -> (→"Speed":cluster{"Numeric":dbl, dbl})  [unwired: 1 in]
        n99 = Build Array (concatenate)(w732, w792, w731, w730, w770, w771, w758, w754, w735, w738, w715, w733, w716, w714) -> (w742:dbl[])
        n100 = Build Array(w735, w715) -> (w739:dbl[])
        n101 = Array Size(array=w742) -> (size(s)=→"size(s)":i32)
        n102 = call "[RT] Array_And_Size.vi"("Select"=enum16{"READ", "WRITE"}."WRITE", "Data In"=w742) -> ()  [unwired: 1 in, 2 out]
        n103 = call "[FGV]Speed.vi"("Select"=enum16{"READ", "WRITE"}."WRITE", "Array"=w739) -> ()  [unwired: 9 in, 1 out]
        n104 = call "[FGV]StopProgram.vi"("Select"=enum16{"READ", "WRITE"}."WRITE", "Flag In"="STOP") -> ()  [unwired: 9 in, 1 out]
        n105 = node-c288() -> ()  [unwired: 1 in, 1 out]
      }
      n106 = timed-loop {
        tunnel: [w294] -> w118
        tunnel: w117 -> [w303]
        timing: w116 -> [_]
        timing-out: [_] -> w115
        stop <- w292 stop-if-true
        n107 = node-c288() -> ()  [unwired: 1 in, 1 out]
        n108 = xnode "FSR Input"() -> ("FSR 1 - Right (B/AI0 (Pin 3))"=w273:dbl)  [unwired: 1 in, 2 out]
        n109 = call "[FGV]IMU.vi"("Select"=enum16{"READ", "WRITE"}."READ") -> ("IMU Out"=w287:dbl[])  [unwired: 1 in]
        n110 = call "[FGV]Speed.vi"("Select"=enum16{"READ", "WRITE"}."READ") -> ("Array 2"=w278:dbl[])  [unwired: 10 in]
        n111 = Greater?(x=w273, y=2.0) -> (0:w271:bool)
        n112 = Index Array(array=w278, index #1=0 ("index")) -> (element #2=w277:dbl)  [unwired: 1 in, 1 out]
        n113 = xnode "One Shot Rising with Input"("input"=w271) -> ("output"=w276:bool)  [unwired: 1 in, 1 out]
        n114 = call "[FGV]HipAngle.vi"("Select"=enum16{"READ", "WRITE"}."READ") -> ("Hip Out"=w291:cluster{dbl, dbl})  [unwired: 10 in]
        n115 = call "[FGV]StopProgram.vi"("Select"=enum16{"READ", "WRITE"}."READ") -> ("Flag Out"=w292:bool)  [unwired: 10 in]
        n116 = Index Array(array=w287, index #1=0 ("index")) -> (element #1=w300:dbl, element #2=w299:dbl, element #3=w298:dbl, element #4=w297:dbl, element #5=w296:dbl, element #6=w295:dbl, element #7=w285:dbl, element #8=w284:dbl, element #9=w283:dbl, element #10=w282:dbl, element #11=w281:dbl, element #12=w280:dbl)  [unwired: 11 in]
        n117 = Unbundle(w291) -> (w286:dbl)  [unwired: 1 out]
        n118 = Boolean To (0,1)(Boolean=w276) -> (0, 1=w275:i16)
        n119 = To Double Precision Float(number=w275) -> (double precision float=w274:dbl)
        n120 = case shown="True" "SEND DATA !!\nLETS GO!" {
          tunnel: w303 -> [w382 w414]
          tunnel: w286 -> [_ w384]
          tunnel: w300 -> [_ w413]
          tunnel: w299 -> [_ w412]
          tunnel: w298 -> [_ w411]
          tunnel: w297 -> [_ w410]
          tunnel: w296 -> [_ w409]
          tunnel: w295 -> [_ w408]
          tunnel: w285 -> [_ w407]
          tunnel: w284 -> [_ w406]
          tunnel: w283 -> [_ w405]
          tunnel: w282 -> [_ w404]
          tunnel: w281 -> [_ w403]
          tunnel: w280 -> [_ w402]
          tunnel: [w382 w401] -> w294
          tunnel: w274 -> [_ w391]
          tunnel: w277 -> [_ w383]
          frame False {
          }
          frame True {
            n121 = Format Into String(format string="%.3f %.3f %.3f %.3f %.3f %.3f %.3f %.3f %.3f %.3f %.3f %.3f %.3f %.3f %.3f", w384, w413, w412, w411, w410, w409, w408, w407, w406, w405, w404, w403, w402, w391, w383) -> (resulting string=w416:string)  [unwired: 2 in, 1 out]
            n122 = call <vilib>:"Space Constant.vi"() -> ("String"=w415:string)
            n123 = Concatenate Strings(w416, w415) -> (w390:string)
            n124 = TCP Write(connection ID=w414, data in=w390) -> (connection ID out=w393:refnum<k5>)  [unwired: 2 in, 2 out]
            n125 = call <vilib>:"Space Constant.vi"() -> ("String"=w398:string)
            n126 = TCP Read(connection ID=w393, bytes to read=20, 7:T28."Immediate" ("mode (standard)")) -> (connection ID out=w401:refnum<k5>, data out=w397:string)  [unwired: 2 in, 1 out]
            n127 = Search/Split String(string=w397, search string/char (-)=w398) -> (substring before match=w392:string, match + rest of string=w399:string)  [unwired: 1 in, 1 out]
            n128 = Search/Split String(string=w399, search string/char (-)=w398, offset (0)=1) -> (substring before match=w400:string)  [unwired: 2 out]
            n129 = Fract/Exp String To Number(string=w392) -> (number=w385:dbl)  [unwired: 3 in, 1 out]
            n130 = call <vilib>:"Trim Whitespace.vi"("string"=w400) -> ("trimmed string"=w389:string)  [unwired: 1 in]
            n131 = Fract/Exp String To Number(string=w389) -> (number=w386:dbl)  [unwired: 3 in, 1 out]
            n132 = Build Array(w385, w386) -> (w388:dbl[])
            n133 = call "[FGV]GP_ML.vi"("Select"=enum16{"READ", "WRITE"}."WRITE", "GP In"=w388) -> ()  [unwired: 9 in, 1 out]
          }
        }
        n134 = node-c288() -> ()  [unwired: 1 in, 1 out]
      }
      n135 = while {
        tunnel: [w706] -> w124
        tunnel: w123 -> [w702]
        stop <- w707 stop-if-true
        n136 = Wait Until Next ms Multiple(millisecond multiple=u32 10 ("millisecond timer value")) -> ()  [unwired: 1 out]
        n137 = call "[RT] Array_And_Size.vi"("Select"=enum16{"READ", "WRITE"}."READ") -> ("Data Out"=w700:dbl[])  [unwired: 2 in, 1 out]
        n138 = Array Size(array=w700) -> (size(s)=w701:i32)
        n139 = for {
          N: w701 -> [_]
          tunnel: w700 -> [w713] mode=indexing
          shift-right: [w711] -> w699
          shift-left: "" -> [w712]
          n140 = Format Into String(initial string=w712, w713) -> (resulting string=w710:string)  [unwired: 2 in, 1 out]
          n141 = Concatenate Strings(w710, " " ("string")) -> (w711:string)
        }
        n142 = Concatenate Strings(w699, "\r") -> (w704:string)
        n143 = call "[FGV]StopProgram.vi"("Select"=enum16{"READ", "WRITE"}."READ") -> ("Flag Out"=w707:bool)  [unwired: 10 in]
        n144 = Write to Text File(file (use dialog)=w702, text=w704) -> (refnum out=w706:refnum<file>)  [unwired: 2 in, 2 out]
      }
      n145 = while {
        tunnel: w120 -> [w432]
        tunnel: [w428] -> w122
        tunnel: w119 -> [w426]
        tunnel: [w424] -> w121
        stop <- w429 stop-if-true
        n146 = flat-sequence {
          tunnel: w432 -> [w442]
          tunnel: [w443] -> w427
          tunnel: w426 -> [w440]
          tunnel: [w438] -> w425
          tunnel: [w454] -> w428
          tunnel: w427 -> [w455]
          tunnel: w425 -> [w448]
          tunnel: [w447] -> w424
          tunnel: [w445] -> w421
          tunnel: [w446] -> w423
          tunnel: [w444] -> w420
          frame #0 {
            n147 = Wait (ms)(milliseconds to wait=u32 7) -> ()  [unwired: 1 out]
            n148 = VISA Write(VISA resource name=w442, write buffer=":84\\n") -> (VISA resource name out=w443:refnum<visa-resource-name>)  [unwired: 1 in, 2 out]
            n149 = VISA Write(VISA resource name=w440, write buffer=":84\\n" ("write buffer 2")) -> (VISA resource name out=w438:refnum<visa-resource-name>)  [unwired: 1 in, 2 out]
          }
          frame #1 {
            n150 = property class="Instr"(reference=w448) -> (reference out=w452:refnum<visa-resource-name>, "Serial Settings:Number of Bytes at Serial Port"=w453:u32)  [unwired: 1 in, 1 out]
            n151 = property class="Instr"(reference=w455) -> (reference out=w459:refnum<visa-resource-name>, "Serial Settings:Number of Bytes at Serial Port"=w460:u32)  [unwired: 1 in, 1 out]
            n152 = VISA Read(VISA resource name=w459, byte count=w460) -> (VISA resource name out=w454:refnum<visa-resource-name>, read buffer=w457:string)  [unwired: 1 in, 2 out]
            n153 = VISA Read(VISA resource name=w452, byte count=w453) -> (VISA resource name out=w447:refnum<visa-resource-name>, read buffer=w450:string)  [unwired: 1 in, 2 out]
            n154 = for {
              N: 6 -> [_]
              tunnel: [w581] -> w456 mode=indexing
              shift-right: [w580] -> _
              shift-left: w457 -> [w579]
              n155 = xnode "Match Regular Expression"("input string"=w579, "regular expression"=",|\\n") -> ("before match"=w581:string, "after match"=w580:string)  [unwired: 4 in, 3 out]
            }
            n156 = for {
              N: 6 -> [_]
              tunnel: [w463] -> w449 mode=indexing
              shift-right: [w462] -> _
              shift-left: w450 -> [w461]
              n157 = xnode "Match Regular Expression"("input string"=w461, "regular expression"=",|\\n") -> ("before match"=w463:string, "after match"=w462:string)  [unwired: 4 in, 3 out]
            }
            n158 = Fract/Exp String To Number(string=w456) -> (number=w446:dbl[])  [unwired: 3 in, 1 out]
            n159 = Fract/Exp String To Number(string=w449) -> (number=w445:dbl[])  [unwired: 3 in, 1 out]
            n160 = Build Array (concatenate)(w446, w445) -> (w444:dbl[])
          }
        }
        n161 = disable-structure shown="Disabled" {
          disable-tunnel: w423 -> [w436 _]
          disable-tunnel: w421 -> [w435 _]
          frame Disabled {
            n162 = Array To Cluster(array=w436) -> (cluster=→"Right IMU":T1)
            n163 = Array To Cluster(array=w435) -> (cluster=→"Trunk IMU":T1)
          }
          frame Enabled {
          }
        }
        n164 = Wait Until Next ms Multiple(millisecond multiple=u32 10) -> ()  [unwired: 1 out]
        n165 = call "[FGV]IMU.vi"("Select"=enum16{"READ", "WRITE"}."WRITE", "IMU In"=w420) -> ()  [unwired: 1 out]
        n166 = call "[FGV]StopProgram.vi"("Select"=enum16{"READ", "WRITE"}."READ") -> ("Flag Out"=w429:bool)  [unwired: 10 in]
      }
      n167 = while {
        i -> [w152]
        stop <- w131 stop-if-true
        w142 = 0.0
        w149 = 50.0 ("y")
        n168 = xnode "FSR Input"() -> ("FSR 1 - Right (B/AI0 (Pin 3))"=w141:dbl, "FSR 2 - Left (B/AI1 (Pin 5))"=w140:dbl)  [unwired: 1 in, 1 out]
        n169 = Wait (ms)(milliseconds to wait=u32 10) -> ()  [unwired: 1 out]
        n170 = Greater?(x=w141, y=2.0) -> (0:w154:bool)
        "R.FSR" <- w154
        n171 = Greater?(x=w140, y=2.0) -> (0:w153:bool)
        "L.FSR" <- w153
        n172 = xnode "One Shot Rising with Input"("input"=w154) -> ("output"=w150:bool)  [unwired: 1 in, 1 out]
        n173 = xnode "One Shot Rising with Input"("input"=w153) -> ("output"=w148:bool)  [unwired: 1 in, 1 out]
        n174 = Multiply(x=w152, y=10) -> (x*y=w135:i32)
        n175 = feedback #7(w142) -> (w144:dbl)
        n176 = Greater?(x=w144, y=w149) -> (0:w146:bool)
        n177 = And(x=w150, y=w146) -> (x .and. y?=w137:bool)
        n178 = feedback #8(w142) -> (w143:dbl)
        n179 = Greater?(x=w143, y=w149) -> (0:w147:bool)
        n180 = And(x=w148, y=w147) -> (x .and. y?=w136:bool)
        n181 = call "[SubV]Gait_Phase_Estimate_R.vi"("Index"=w135, "Hill Contact"=w137) -> ("GP"=w138:dbl, "Cadence"=w139:dbl)
        n182 = feedback-in #7(w138) -> ()
        n183 = call "[SubV]Gait_Phase_Estimate_L.vi"("Index"=w135, "Hill Contact"=w136) -> ("GP"=w133:dbl, "Cadence"=w134:dbl)
        n184 = feedback-in #8(w133) -> ()
        n185 = Build Array(w138, w133, w139, w134, w141, w140) -> (w130:dbl[])
        n186 = call "[FGV]StopProgram.vi"("Select"=enum16{"READ", "WRITE"}."READ") -> ("Flag Out"=w131:bool)  [unwired: 10 in]
        n187 = call "[FGV]GaitPhase.vi"("Select"=enum16{"READ", "WRITE"}."WRITE", "GP In"=w130) -> ()  [unwired: 9 in, 1 out]
      }
      n188 = node-c288(w115) -> ()  [unwired: 1 out]
      n189 = TCP Close Connection(connection ID=w118) -> ()  [unwired: 2 in, 2 out]
      n190 = VISA Close(VISA resource name=w121) -> ()  [unwired: 1 in, 1 out]
      n191 = VISA Close(VISA resource name=w122) -> ()  [unwired: 1 in, 1 out]
      n192 = node-c288(w127) -> ()  [unwired: 1 out]
    }
    frame #2 {
      n193 = call <vilib>:"Close.vi"("SPI Ref In"=w1117) -> ()  [unwired: 10 in, 1 out]
      n194 = Close File(refnum=w1116) -> ()  [unwired: 1 in, 2 out]
    }
    frame #3 {
      n195 = call <vilib>:"Reset myRIO.vi"() -> ()  [unwired: 11 in, 1 out]
    }
  }
